vi "Close.vi"(8 "error in":errorcluster, 11 "Voltage Control in":refnum<class "Voltage Control.lvclass">) -> (0 "error out":errorcluster, 3 "Voltage Control out":refnum<class "Voltage Control.lvclass">)   [LabVIEW 2023, in "Voltage Control.lvclass"]
uses:
  Voltage Control.lvclass
  Voltage Control.lvclass/Voltage Control.ctl
  <vilib>/ADAS Replay HIL/AdasHilServices/AdasHilChannelServices.lvlib
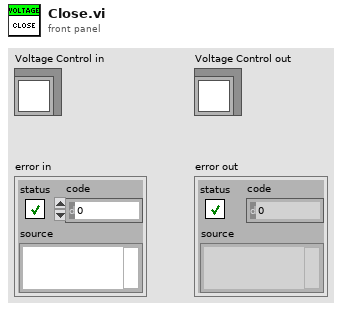
[diagram p1: front panel]
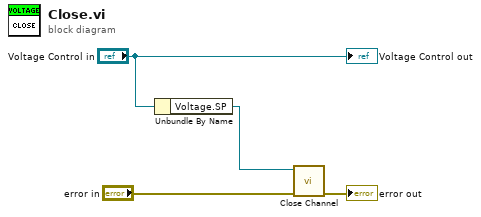
[diagram p0: block diagram]
diagram:
  n1 = Unbundle By Name("Voltage Control in") -> ("Voltage.SP"=w2:refnum<k21>)
  n2 = call <vilib>:"Close Channel.vi"("error in"="error in", "ADAS HIL Channel"=w2) -> ("error out"=→"error out":errorcluster)  [unwired: 9 in]
  "Voltage Control out" <- "Voltage Control in"
